vi "Create Status Events.vi"(8 "error in (no error)":errorcluster, 11 "XY Stage Data Class in":refnum<class "XY Stage Data Class.lvclass">) -> (0 "error out":errorcluster, 3 "XY Stage Data Class out":refnum<class "XY Stage Data Class.lvclass">)   [LabVIEW 2022 SP3, in "XY Stage Data Class.lvclass"]
uses:
  XY Stage Data Class.lvclass
  XY Position.ctl
  Moving.ctl
  Homed.ctl
  Current Speed.ctl
  Acceleration.ctl
  Speed.ctl
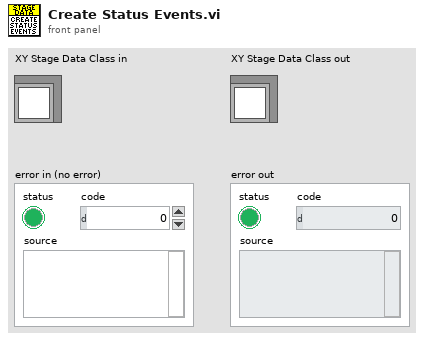
[diagram p1: front panel]
types:
  T1 = typedef "XY Stage Data Class.lvclass/Speed.ctl" = cluster{"X-Speed":dbl, "Y-Speed":dbl}
  T2 = typedef "XY Stage Data Class.lvclass/Acceleration.ctl" = cluster{"X Acceleration":dbl, "Y Acceleration":dbl}
  T3 = typedef "XY Stage Data Class.lvclass/Current Speed.ctl" = cluster{"X Current Speed":dbl, "Y Current Speed":dbl}
  T4 = typedef "XY Stage Data Class.lvclass/Homed.ctl" = cluster{"X Homed":bool, "Y Homed":bool}
  T5 = typedef "XY Stage Data Class.lvclass/Moving.ctl" = cluster{"X Moving":bool, "Y Moving":bool}
  T6 = typedef "XY Stage Data Class.lvclass/XY Position.ctl" = cluster{"Current Position X":dbl, "Current Position Y":dbl}
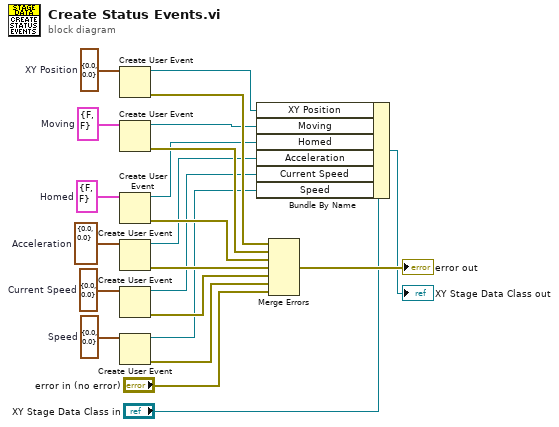
[diagram p0: block diagram]
diagram:
  w3 = T1 {"X-Speed"=0.0, "Y-Speed"=0.0}  # Speed
  w6 = T2 {"X Acceleration"=0.0, "Y Acceleration"=0.0}  # Acceleration
  w5 = T3 {"X Current Speed"=0.0, "Y Current Speed"=0.0}  # Current Speed
  w7 = T4 {"X Homed"=FALSE, "Y Homed"=FALSE}  # Homed
  w8 = T5 {"X Moving"=FALSE, "Y Moving"=FALSE}  # Moving
  w9 = T6 {"Current Position X"=0.0, "Current Position Y"=0.0}  # XY Position
  n1 = Create User Event(user event datatype=w9) -> (user event=w15:refnum<user-event>, error out=w16:errorcluster)  [unwired: 1 in]
  n2 = Create User Event(user event datatype=w8) -> (user event=w14:refnum<user-event>, error out=w17:errorcluster)  [unwired: 1 in]
  n3 = Create User Event(user event datatype=w7) -> (user event=w13:refnum<user-event>, error out=w18:errorcluster)  [unwired: 1 in]
  n4 = Create User Event(user event datatype=w6) -> (user event=w12:refnum<user-event>, error out=w19:errorcluster)  [unwired: 1 in]
  n5 = Create User Event(user event datatype=w5) -> (user event=w11:refnum<user-event>, error out=w20:errorcluster)  [unwired: 1 in]
  n6 = Create User Event(user event datatype=w3) -> (user event=w2:refnum<user-event>, error out=w1:errorcluster)  [unwired: 1 in]
  n7 = Bundle By Name(cluster="XY Stage Data Class in", "XY Position"=w15, "Moving"=w14, "Homed"=w13, "Acceleration"=w12, "Current Speed"=w11, "Speed"=w2) -> (→"XY Stage Data Class out":refnum<class "XY Stage Data Class.lvclass">)
  n8 = Merge Errors(w16, w17, w18, w19, w20, w1, "error in (no error)") -> (→"error out":errorcluster)
